vi "DEMO.vi"() -> ()   [LabVIEW 2012, in "Dictionary.lvclass"]
uses:
  Dictionary.lvclass
  Dictionary.lvclass/Dictionary.ctl
panel:
  out "Values Array 2":string[](array[string])
  out "Keys Array 2":string[](array[string])
  out "Key Exist?":bool
  out "Value":string
  out "Values Array":string[](array[string])
  out "Keys Array":string[](array[string])
  in  "组合框":string(combo)
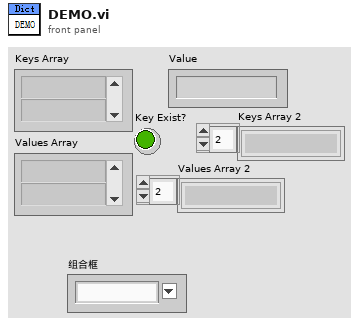
[diagram p1: front panel]
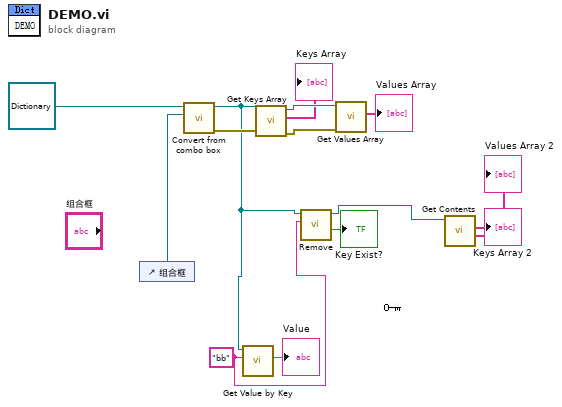
[diagram p0: block diagram]
diagram:
  w5 = "bb" ("Key")
  n1 = control-ref of="组合框"() -> (w8:refnum<vi>)
  n2 = call "Convert from combo box.vi"("CmbBox Ref"=w8, "Dictionary In"=refnum<class "Dictionary.lvclass"> refnum) -> ("error out"=w13:errorcluster, "Dictionary Out"=w6:refnum<class "Dictionary.lvclass">)  [unwired: 8 in]
  n3 = call "Get Value by Key.vi"("Key"=w5, "Dictionary In"=w6) -> ("Value"=→"Value":string)  [unwired: 6 in, 3 out]
  n4 = call "Get Keys Array.vi"("error in"=w13, "Dictionary in"=w6) -> ("error out"=w11:errorcluster, "Keys Array"=→"Keys Array":string[], "Dictionary out"=w12:refnum<class "Dictionary.lvclass">)  [unwired: 7 in]
  n5 = call "Remove.vi"("Key"=w5, "Dictionary In"=w6) -> ("Key Exist?"=→"Key Exist?":bool, "Dictionary Out"=w3:refnum<class "Dictionary.lvclass">)  [unwired: 6 in, 2 out]
  n6 = call "Get Values Array.vi"("error in"=w11, "Dictionary in"=w12) -> ("Values Array"=→"Values Array":string[])  [unwired: 7 in, 2 out]
  n7 = call "Get Contents.vi"("Dictionary In"=w3) -> ("Values Array"=→"Values Array 2":string[], "Keys Array"=→"Keys Array 2":string[])  [unwired: 7 in, 2 out]
